vi "set_exposure.vi"(7 "error in (no error)":errorcluster, 8 "cam ID":u32, 9 "exposure":dbl, 10 "Session in":refnum<k35>) -> (0 "error out":errorcluster, 1 "true FPS":dbl, 2 "true exposure":dbl, 3 "session out":refnum<k35>)   [LabVIEW 2022 SP3]
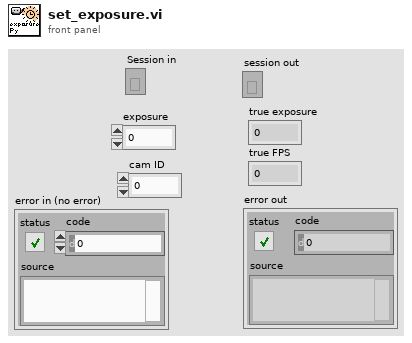
[diagram p1: front panel]
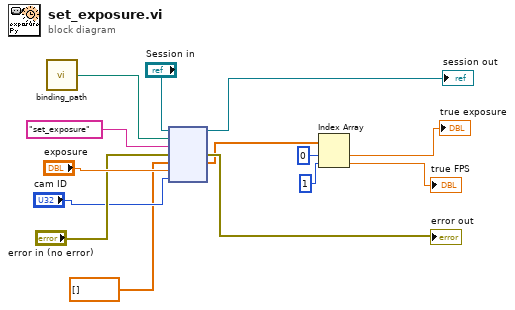
[diagram p0: block diagram]
diagram:
  n1 = call "binding_path.vi"() -> ("appended path"=w11:path)
  n2 = node("Session in", w11, "set_exposure" ("function name"), "error in (no error)", dbl[] [], "exposure", "cam ID") -> (→"session out":refnum<k35>, →"error out":errorcluster, w5:dbl[])  [unwired: 2 in, 2 out]
  n3 = Index Array(array=w5, index #1=0 ("index"), index #2=1 ("index")) -> (element #1=→"true exposure":dbl, element #2=→"true FPS":dbl)
